vi "CIPC U8 Array FIFO.vi"() -> (3 "CIF_CIPC_Fifo_U8.lvclass":refnum<class "CIF_CIPC_Fifo_U8.lvclass">)   [LabVIEW 2021, in "CIF_CIPC_Fifo_U8.lvclass"]
uses:
  CIF_CIPC_Fifo_U8.lvclass
  CIF_CIPC_Fifo_U8.lvclass/CIF_CIPC_Fifo_U8.ctl
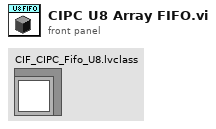
[diagram p1: front panel]
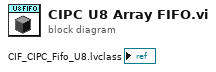
[diagram p0: block diagram]
diagram:
